vi "Get Relay Position.vi"(8 "error in (no error)":errorcluster, 10 "relay name":string, 11 "session in":T2) -> (0 "error out":errorcluster, 2 "position":T1=10 items=["Open"=10, "Closed"=11], 3 "session out":T2)   [LabVIEW 2020, in "SLSC Switch.lvlib"]
doc: "Returns the relay position for the relay specified in <B>relay name</B>."
uses:
  <vilib>/SLSC_Switch/SLSC Switch.lvlib
  nislscsl.dll
  <vilib>/userdefined/High Color/SLSC_Switch/nislscslSession.ctl
  <vilib>/SLSC_Switch/Relay Position.ctl
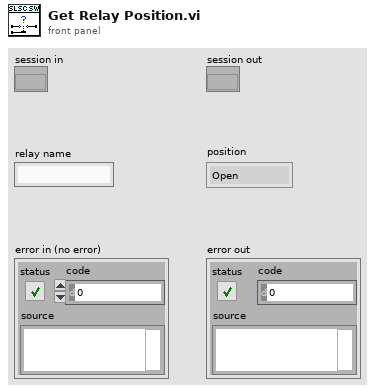
[diagram p1: front panel]
types:
  T1 = typedef "SLSC Switch.lvlib/Relay Position.ctl" = i32
  T2 = typedef "nislscslSession.ctl" = refnum<k20>
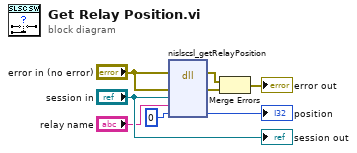
[diagram p0: block diagram]
diagram:
  n1 = dll-call lib="nislscsl.*" fn="nislscsl_getRelayPosition"(error in="error in (no error)", "errorCluster"="error in (no error)", "sessionHandle"="session in", "relayName"="relay name", "position"=0) -> (error out=w8:errorcluster, "errorCluster"=w7:errorcluster, "position"=→"position":i32)  [unwired: 5 in, 1 out]
  n2 = Merge Errors(w8, w7) -> (→"error out":errorcluster)
  "session out" <- "session in"
